vi "TimingTest.vi"() -> ()   [LabVIEW 2019]
uses:
  <vilib>/Analysis/Matrix/Numeric/Multiply/Multiply - RM,RM.vi
  <vilib>/Analysis/Matrix/NI_Matrix.lvlib
panel:
  out "time":u32
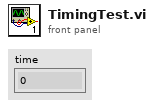
[diagram p1: front panel]
types:
  T1 = typedef "NI_Matrix.lvlib/RealMatrix.ctl" = dbl[][]
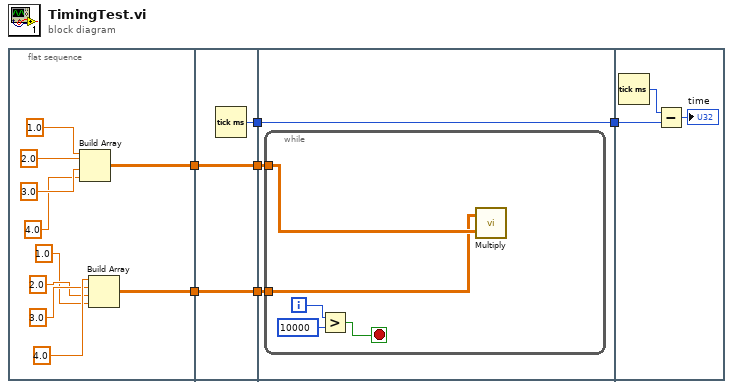
[diagram p0: block diagram]
diagram:
  n1 = flat-sequence {
    tunnel: [w8] -> w3
    tunnel: [w7] -> w1
    tunnel: [w19] -> w5
    tunnel: [w18] -> w4
    tunnel: w3 -> [w18]
    tunnel: [w17] -> w2
    tunnel: w1 -> [w17]
    tunnel: [w22] -> w6
    tunnel: w5 -> [w22]
    tunnel: w4 -> [w21]
    tunnel: w2 -> [w20]
    tunnel: w6 -> [w29]
    frame #0 {
      n2 = Build Array(1.0, 2.0, 3.0, 4.0) -> (w8:T1)
      n3 = Build Array(4.0, 3.0, 2.0, 1.0) -> (w7:T1)
    }
    frame #1 {
      n4 = Tick Count (ms)() -> (millisecond timer value=w19:u32)
    }
    frame #2 {
      n5 = while {
        tunnel: w21 -> [w24]
        tunnel: w20 -> [w23]
        i -> [w27]
        stop <- w25 stop-if-true
        n6 = Greater?(x=w27, y=10000) -> (0:w25:bool)
        n7 = call-poly <vilib>:"Multiply.vi"("Real Matrix B"=w24, "Real Matrix A"=w23) -> ()  [unwired: 1 out]
      }
    }
    frame #3 {
      n8 = Tick Count (ms)() -> (millisecond timer value=w30:u32)
      n9 = Subtract(x=w30, y=w29) -> (x-y=→"time":u32)
    }
  }
